vi "Streaming 2955 simple.vi"() -> ()   [LabVIEW 2021]
doc: "Acquires data from the Rx ports and streams the data to the host while receiving data from the host and generating the resulting waveform at the Tx ports of the NI USRP 294x/295x device. Use this VI as a template for the Simple NI-USRP Streaming sample project."
uses:
  <instrlib>/_niInstr/Register Bus/v1/FPGA/Public/Read Cmd Data.ctl
  <vilib>/Platform/TimedLoop/XDataNode/timing_clust.ctl
  <vilib>/Platform/TimedLoop/XDataNode/nitl_modes.ctl
  <vilib>/Platform/TimedLoop/XDataNode/wakeup.ctl
  <vilib>/rvi/Emulation/niFpgaSctlEmulationGetInTimedLoop.vi
  <vilib>/rvi/Emulation/niFpgaEmulationReportErrorSimple.vi
  <vilib>/rvi/Emulation/niFpgaGetClockAttributes.vi
  <vilib>/rvi/Emulation/niFpgaCriticalErrorInLSC.vi
  <vilib>/rvi/eio/common/nirviEmuTemplateMethod_errors.vi
  <instrlib>/_niInstr/DSP/v1/FPGA/Public/Sub VIs/Data Conversion/I16 to IQ - 1 spc - S18.1.vi
  <instrlib>/_niInstr/Basic Elements/v1/FPGA/Private/Count Up U32.vi
  <vilib>/rvi/interface/RandomDataEmulation/nirviRandomDataMultiElementFPGAFIFO.vi
  <instcachedir>/0/nirviRandomDataMultiElementFPGAFIFO_3E9965BA1FAD4E7B8DABA31768A09B1F.lvgen/nirviRandomDataMultiElementFPGAFIFO_3E9965BA1FAD4E7B8DABA31768A09B1F_003.vi
  <vilib>/rvi/interface/RandomDataEmulation/niFpgaRandomDataHandleErrors.vi
  <vilib>/Platform/TimedLoop/XDataNode/XDataNode.xnode
  <vilib>/eio/EIONode/EIONode.xnode
  <vilib>/rvi/DataTransferAndStorage/Container/XNode/niFpgaContainer.xnode
  <vilib>/rvi/interface/RandomDataEmulation/nirviRandomDataFpgaMultiElementTemplate.vi
  <vilib>/Platform/TimedLoop/XDataNode/XDNodeRunTimeDep.lvlib
  <instrlib>/niUsrpRio/Config/v1/FPGA/niUsrpRio Config v1 FPGA.lvlib
  <instrlib>/_niInstr/DSP/v1/FPGA/niInstr DSP v1 FPGA.lvlib
  <instrlib>/_niInstr/Basic Elements/v1/FPGA/niInstr Basic Elements v1 FPGA.lvlib
  <instrlib>/_niInstr/Register Bus/v1/FPGA/niInstr Register Bus v1 FPGA.lvlib
panel:
  in  "LED/RF /RX2":enum8{"Off", "Green"}(ring)
  in  "LED/RF /RX1":enum8{"Off", "Green", "Red", "Amber"}(ring)
  out "data sent":u32
  out "number of overflows":u64[](array[numeric])
  out "lost sampels":u32
  in  "DSP params":T1(array[cluster])=[{"output sample rate"=0.0, "delay"=0.0, "frequency shift"=0.0, "phase"=0.0}, {"output sample rate"=0.0, "delay"=0.0, "frequency shift"=0.0, "phase"=0.0}, {"output sample rate"=0.0, "delay"=0.0, "frequency shift"=0.0, "phase"=0.0}, {"output sample rate"=0.0, "delay"=0.0, "frequency shift"=0.0, "phase"=0.0}] {"frequency shift" format="%#.48g"}
  in  "reset":bool
  in  "RF 1/Tx/Enable":bool
  in  "RF 1/Rx/Enable":bool
  in  "RF 0/Tx/Enable":bool
  in  "RF 0/Rx/Enable":bool
  in  "reg.host read.go rcvd 0":bool
  out "reg.notify host.go 0":bool
  in  "reg.notify host.go rcvd 0":bool
  out "reg.host read.data 0":T2
  in  "reg.reset 0":bool
  # "FPGA utilization"
  # "USRP RIO Simple Streaming FPGA"
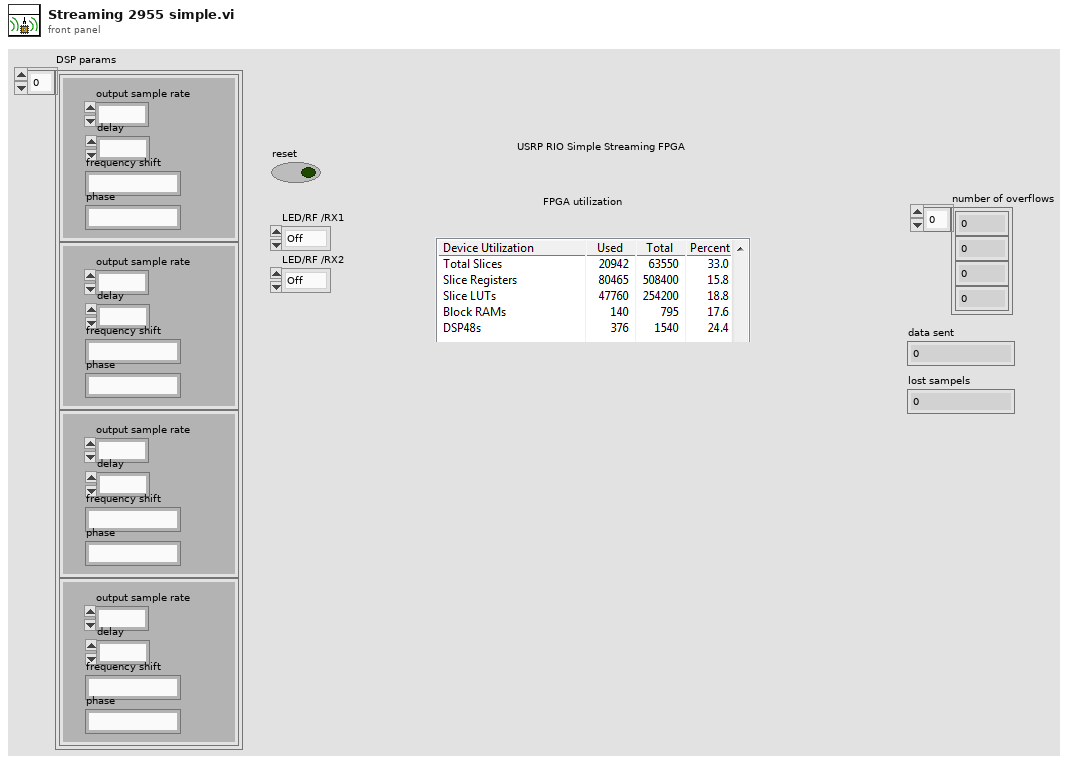
[diagram p1: front panel]
types:
  T1 = cluster{"output sample rate":fxp<+,48,1>, "delay":fxp<+/-,16,0>, "frequency shift":fxp<+/-,48,0>, "phase":fxp<+/-,21,0>}[]
  T2 = typedef "niInstr Register Bus v1 FPGA.lvlib/Read Cmd Data.ctl" = cluster{"go":bool, "data":u32}
  T3 = typedef "XDNodeRunTimeDep.lvlib/timing_clust.ctl" = cluster{"Expected End [f-1]":u64, "Actual End [f-1]":u64, "Finished Late? [f-1]":bool, "Expected End [i-1]":u64, "Actual End [i-1]":u64, "Finished Late? [i-1]":bool, "Expected Start [i]":u64, "Actual Start [i]":u64, "Expected Start [f]":u64, "Actual Start [f]":u64, "Source Name":string, "Structure Name":string, "Period":i64, "Deadline":i64, "Offset":i64, "Start":i64, "Priority":i32, "Timeout":i32, "Mode":T4, "Wakeup Reason":T5, "Error":errorcluster, "Source Type":string, "Secondary Source Type":string, "Global End Time":u64, "Global Start Time":u64, "Frame Duration":u64, "Iteration Duration":u64, "Assigned CPU":i32, "I/O Scan Engine Mode":u32}
  T4 = typedef "XDNodeRunTimeDep.lvlib/nitl_modes.ctl" = enum32{"No Change", "Process missed periods, maintain original phase", "Discard missed periods, maintain original phase", "Process missed periods, ignore original phase", "Discard missed periods, ignore original phase"}
  T5 = typedef "XDNodeRunTimeDep.lvlib/wakeup.ctl" = enum32{"Normal", "Aborted", "Asynchronous wakeup", "Timing source error", "Timed loop error", "Timeout"}
  T6 = cluster{"output sample rate":fxp<+,48,1>, "delay":fxp<+/-,16,0>, "frequency shift":fxp<+/-,48,0>, "phase":fxp<+/-,21,0>}
  T7 = typedef "niInstr DSP v1 Shared.lvlib/IQ Data.ctl" = cluster{"I":fxp<+/-,18,1>, "Q":fxp<+/-,18,1>, "overflow":bool}
  T8 = cluster{"DAC FIFO Reset":refnum<k21>, "RF 0 Rx Swap IQ":refnum<k21>, "RF 0 Rx Negate I":refnum<k21>, "RF 0 Rx Negate Q":refnum<k21>, "RF 0 Rx Data Valid":refnum<k21>, "RF 0 Rx Data Ever Invalid":refnum<k21>, "clear RF 0 Rx Data Ever Invalid":refnum<k21>, "RF 0 Tx Swap IQ":refnum<k21>, "RF 0 Tx Negate I":refnum<k21>, "RF 0 Tx Negate Q":refnum<k21>, "RF 1 Rx Swap IQ":refnum<k21>, "RF 1 Rx Negate I":refnum<k21>, "RF 1 Rx Negate Q":refnum<k21>, "RF 1 Rx Data Valid":refnum<k21>, "RF 1 Rx Data Ever Invalid":refnum<k21>, "clear RF 1 Rx Data Ever Invalid":refnum<k21>, "RF 1 Tx Swap IQ":refnum<k21>, "RF 1 Tx Negate I":refnum<k21>, "RF 1 Tx Negate Q":refnum<k21>}
  T9 = typedef "niUsrpRio Synchronization v1 FPGA.lvlib/Resources.ctl" = cluster{"master":refnum<k21>, "meas.enable":refnum<k21>, "meas.ready":refnum<k21>, "meas.reset":refnum<k21>, "meas.arm":refnum<k21>, "meas.valid":refnum<k21>, "meas.value":refnum<k21>, "meas.oversample factor":refnum<k21>, "cptr":refnum<k21>, "cptr.adjust":refnum<k21>, "cptr.period":refnum<k21>}
  T10 = typedef "niUsrpRio Time v1 FPGA.lvlib/Time Resources.ctl" = cluster{"reset":refnum<k21>, "time":refnum<k21>, "time.previous cptr":refnum<k21>, "new time":refnum<k21>, "new time.when":refnum<k21>, "new time.set":refnum<k21>, "which edge of ref":refnum<k21>, "pps source":refnum<k21>, "internal pps period":refnum<k21>}
  T11 = typedef "niUsrpRio Time v1 FPGA.lvlib/Future Event Resources.ctl" = cluster{"reset":refnum<k21>, "future event.time":refnum<k21>, "future event.ready":refnum<k21>, "future event.set":refnum<k21>, "future event.clear":refnum<k21>, "future event.set in past":refnum<k21>}
  T12 = cluster{"time.resources":T10, "future event.resources":T11, "future event.resources":T11, "future event.resources":T11}
  T13 = typedef "Clock Cross Resources.ctl" = cluster{"register instruction":refnum<k21>, "read completion":refnum<k21>}
  T14 = typedef "niInstr Register Bus v1 FPGA.lvlib/Register Instruction.ctl" = cluster{"subsystem":u8, "address":u16, "data":u32, "valid":bool, "read":bool}
  T15 = typedef "niInstr Register Bus v1 FPGA.lvlib/Read Completion.ctl" = cluster{"data":u32, "valid":bool}
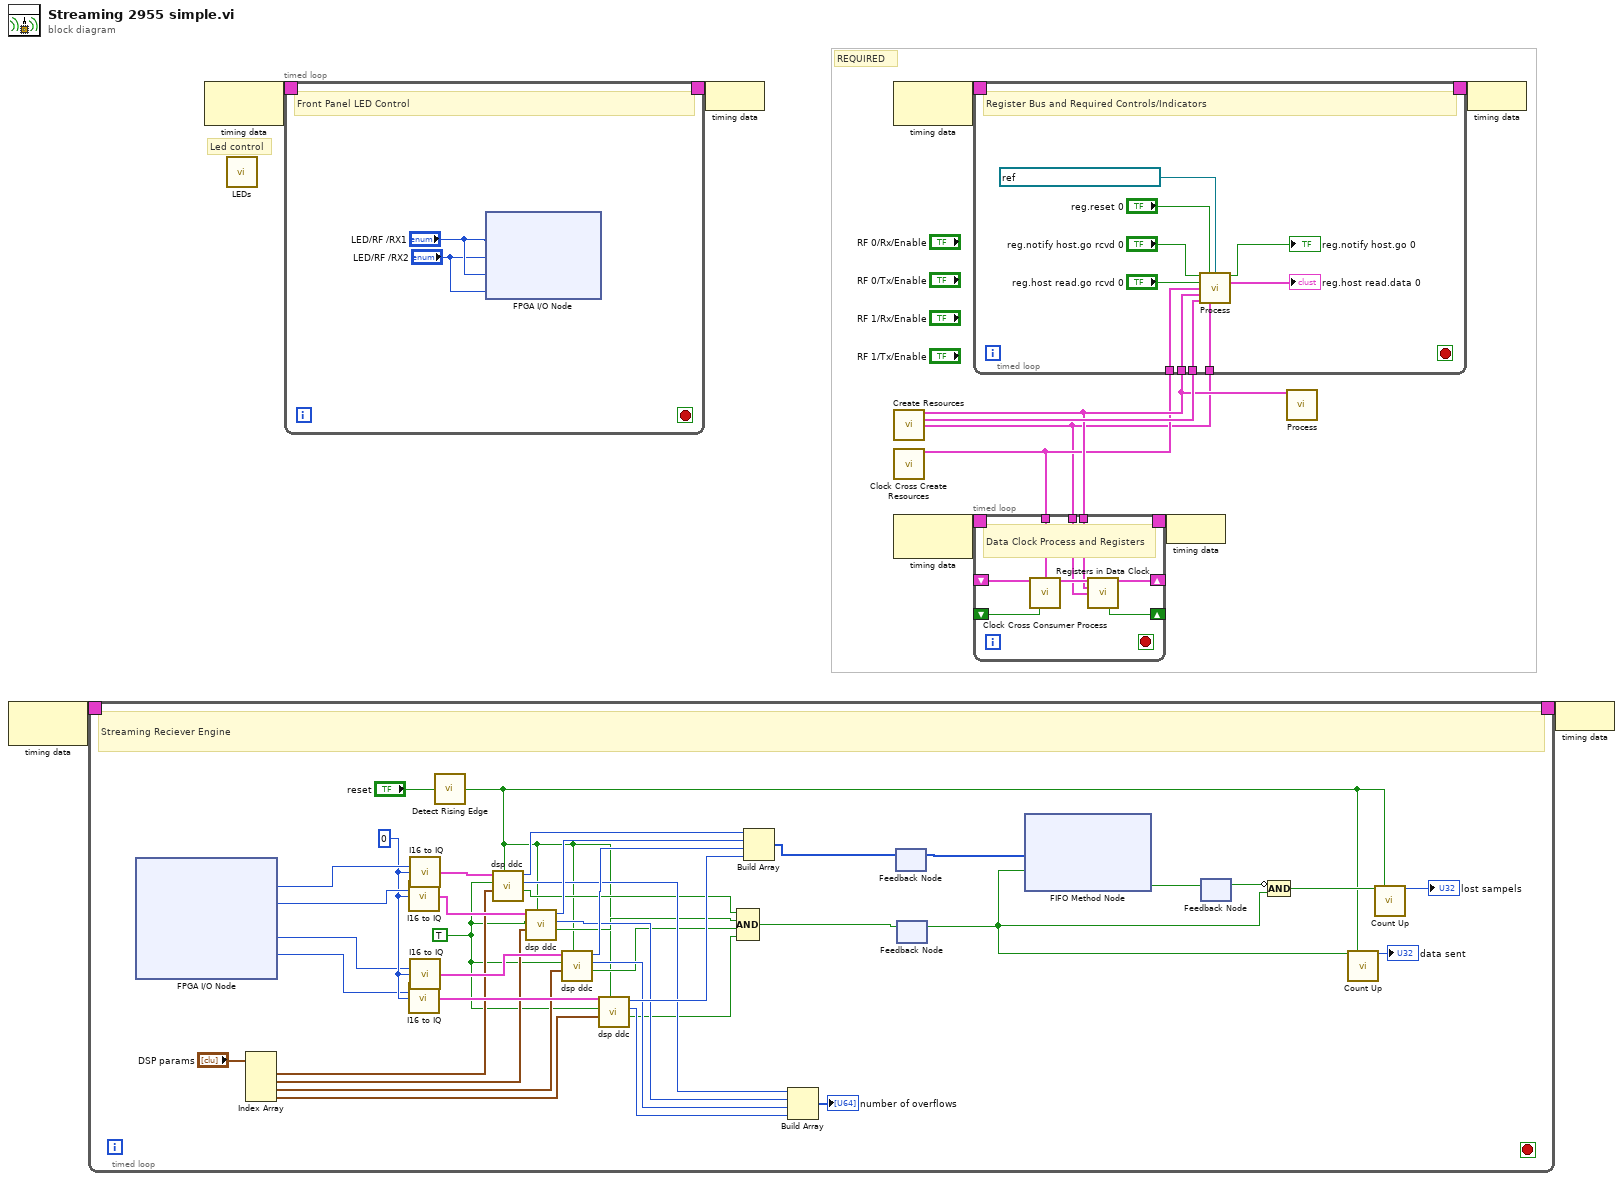
[diagram p0: block diagram]
diagram:
  # "Led control"
  # "REQUIRED"
  n1 = node-c288() -> (w10:T3)  [unwired: 1 in]
  n2 = timed-loop "Streaming Transceiver Engine" {
    timing: w10 -> [_]
    timing-out: [_] -> w9
    stop <- _ stop-if-true
    w17 = TRUE ("input valid")
    w47 = i16 0 ("Q")
    # "Streaming Reciever Engine"
    n3 = xnode "FPGA I/O Node"() -> ("RF 0/Rx/Rx1"=w49:i16, "RF 0/Rx/Rx2"=w50:i16, "RF 1/Rx/Rx1"=w46:i16, "RF 1/Rx/Rx2"=w45:i16)  [unwired: 6 in, 8 out]
    n4 = Index Array(array="DSP params") -> (element #1=w41:T6, element #2=w40:T6, element #3=w39:T6, element #4=w38:T6)  [unwired: 4 in]
    n5 = call-poly <instrlib>:"I16 to IQ.vi"("I"=w50, "Q"=w47) -> ("IQ"=w48:T7)  [unwired: 13 in]
    n6 = call-poly <instrlib>:"I16 to IQ.vi"("I"=w45, "Q"=w47) -> ("IQ"=w43:T7)  [unwired: 13 in]
    n7 = call-poly <instrlib>:"I16 to IQ.vi"("I"=w49, "Q"=w47) -> ("IQ"=w51:T7)  [unwired: 13 in]
    n8 = call-poly <instrlib>:"I16 to IQ.vi"("I"=w46, "Q"=w47) -> ("IQ"=w44:T7)  [unwired: 13 in]
    n9 = call <instrlib>:"Detect Rising Edge.vi"("signal"="reset") -> ("edge detected"=w15:bool)  [unwired: 14 in]
    n10 = call "dsp ddc.vi"("reset"=w15, "DDC prams"=w41, "input valid"=w17, "data in"=w51) -> ("output valid"=w18:bool, "number of overflows"=w24:u64, "data out"=w37:u32)  [unwired: 5 in]
    n11 = call "dsp ddc.vi"("reset"=w15, "DDC prams"=w40, "input valid"=w17, "data in"=w48) -> ("output valid"=w19:bool, "number of overflows"=w25:u64, "data out"=w36:u32)  [unwired: 5 in]
    n12 = call "dsp ddc.vi"("reset"=w15, "DDC prams"=w39, "input valid"=w17, "data in"=w44) -> ("output valid"=w20:bool, "number of overflows"=w26:u64, "data out"=w35:u32)  [unwired: 5 in]
    n13 = call "dsp ddc.vi"("reset"=w15, "DDC prams"=w38, "input valid"=w17, "data in"=w43) -> ("output valid"=w21:bool, "number of overflows"=w27:u64, "data out"=w34:u32)  [unwired: 5 in]
    n14 = Compound Arithmetic op=AND(w18, w19, w20, w21) -> (w14:bool)
    n15 = Build Array(w37, w36, w35, w34) -> (w33:u32[])
    n16 = Build Array(w24, w25, w26, w27) -> (→"number of overflows":u64[])
    n17 = feedback-in #1(w33) -> ()
    n18 = feedback #1() -> (w32:u32[])  [unwired: 1 in]
    n19 = feedback #2() -> (w13:bool)  [unwired: 1 in]
    n20 = feedback-in #2(w14) -> ()
    n21 = xnode ("FIFO Method Node")("Element"=w32, "Input Valid"=w13) -> ("Ready for Input"=w31:bool)  [unwired: 1 in, 1 out]
    n22 = feedback #3() -> (w30:bool)  [unwired: 1 in]
    n23 = feedback-in #3(w31) -> ()
    n24 = Compound Arithmetic op=AND(invert w30, w13) -> (w29:bool)
    n25 = call-poly <instrlib>:"Count Up.vi"("increment"=w13, "reset"=w15) -> ("count out"=→"data sent":u32)  [unwired: 13 in]
    n26 = call-poly <instrlib>:"Count Up.vi"("increment"=w29, "reset"=w15) -> ("count out"=→"lost sampels":u32)  [unwired: 13 in]
  }
  n27 = node-c288() -> (w2:T3)  [unwired: 1 in]
  n28 = call "LEDs.vi"() -> ()  [unwired: 1 in]
  n29 = timed-loop {
    timing: w2 -> [_]
    timing-out: [_] -> w1
    stop <- _ stop-if-true
    # "Front Panel LED Control"
    n30 = xnode "FPGA I/O Node"("LED/RF 0/RX1"="LED/RF /RX1", "LED/RF 0/RX2"="LED/RF /RX2", "LED/RF 1/RX1"="LED/RF /RX1", "LED/RF 1/RX2"="LED/RF /RX2") -> ()  [unwired: 4 in, 4 out]
  }
  n31 = node-c288(w1) -> ()
  n32 = node-c288() -> (w12:T3)  [unwired: 1 in]
  n33 = call "Create Resources.vi"() -> ("config.resources"=w5:T8, "sync.resources"=w8:T9, "time.resources"=w3:T12)  [unwired: 13 in]
  n34 = call "Clock Cross Create Resources.vi"() -> ("resources"=w4:T13)  [unwired: 15 in]
  n35 = node-c288() -> (w7:T3)  [unwired: 1 in]
  n36 = timed-loop "Register Bus and Required Controls/Indicators" {
    timing: w12 -> [_]
    timing-out: [_] -> w11
    tunnel: w5 -> [w60]
    tunnel: w8 -> [w59]
    tunnel: w3 -> [w58]
    tunnel: w4 -> [w61]
    stop <- _ stop-if-true
    # "Register Bus and Required Controls/Indicators"
    n37 = call <instrlib>:"Process.vi"("reg.notify host.go rcvd"="reg.notify host.go rcvd 0", "reg.reset"="reg.reset 0", "reg.instruction fifo"=refnum<k21> "reg.host instruction fifo 0" ("reg.host instruction fifo"), "reg.host read.go rcvd"="reg.host read.go rcvd 0", "clock cross resources"=w61, "config.resources"=w60, "sync.resources"=w59, "time.resources"=w58) -> ("reg.notify host.go"=→"reg.notify host.go 0":bool, "reg.host read.data"=→"reg.host read.data 0":T2)  [unwired: 6 in]
  }
  n38 = timed-loop {
    timing: w7 -> [_]
    timing-out: [_] -> w6
    shift-right: [w76] -> _
    shift-left: _ -> [w73]
    shift-right: [w75] -> _
    shift-left: _ -> [w74]
    tunnel: w5 -> [w72]
    tunnel: w4 -> [w71]
    tunnel: w3 -> [w70]
    stop <- _ stop-if-true
    # "Data Clock Process and Registers"
    n39 = call "Clock Cross Consumer Process.vi"("read completion"=w73, "resources"=w71, "ready for output"=w74) -> ("register instruction"=w77:T14)  [unwired: 12 in]
    n40 = call "Registers in Data Clock.vi"("register instruction"=w77, "config.resources"=w72, "time.resources"=w70) -> ("read completion out"=w76:T15, "ready for input"=w75:bool)  [unwired: 11 in]
  }
  n41 = node-c288(w6) -> ()
  n42 = call <instrlib>:"Process.vi"("resources"=w5) -> ()  [unwired: 15 in]
  n43 = node-c288(w11) -> ()
  n44 = node-c288(w9) -> ()
